vi "PID Line Follower.vi"(6 "K_i":sgl=0.01, 7 "Port (Gyro)":T1 items=["Port 1", "Port 2", "Port 3", "Port 4"], 8 "K_p":sgl=0.7, 9 "Previous integral\nerror":sgl, 10 "Target reflection":sgl=42.0, 11 "EV3 in":T2) -> (1 "New integral":sgl, 2 "Total error":sgl, 3 "EV3 out":T2)   [LabVIEW 2016]
uses:
  <vilib>/NXT/Subs/LVHSConnector.ctl
  <vilib>/NXT/LegoClasses/BrickReference/BrickReference.lvclass
  <vilib>/NXT/Block Support/NXT_InputPort.ctl
  <vilib>/NXT/Dual Mode Library/Sensors/EV3_Color_Reflect.vi
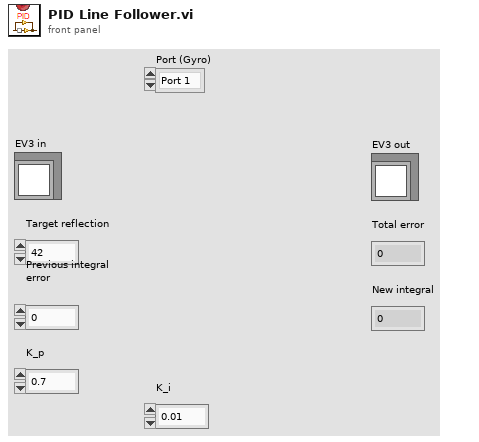
[diagram p1: front panel]
types:
  T1 = typedef "NXT_InputPort.ctl" = u32
  T2 = typedef "LVHSConnector.ctl" = refnum<class "BrickReference.lvclass">
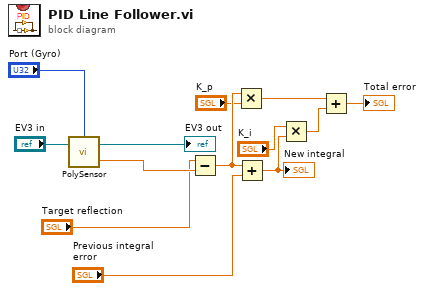
[diagram p0: block diagram]
diagram:
  n1 = call-poly <vilib>:"PolySensor.vi"("NXT/EV3"="EV3 in", "Port (Port 1)"="Port (Gyro)") -> ("Scaled Value"=w2:sgl, "NXT/EV3"=→"EV3 out":T2)  [unwired: 1 in]
  n2 = Subtract(x="Target reflection", y=w2) -> (x-y=w9:sgl)
  n3 = Multiply(x=w9, y="K_p") -> (x*y=w7:sgl)
  n4 = Add(x=w9, y="Previous integral\nerror") -> (x+y=w5:sgl)
  "New integral" <- w5
  n5 = Multiply(x="K_i", y=w5) -> (x*y=w8:sgl)
  n6 = Add(x=w7, y=w8) -> (x+y=→"Total error":sgl)
